vi "Init Incoming Single Point Signals.vi"(8 "error in":errorcluster, 11 "Incoming Single Point Configuraiton":T1 {"Channel Pairs"."Chan Refs" format="%.0x"}) -> (0 "error out":errorcluster, 3 "Incoming Single Point Configuraiton":T5 {"Channel Pairs"."Chan Refs" format="%.0x"})   [LabVIEW 2013, in "J1939 Addon Engine.lvlib"]
uses:
  J1939 Addon Engine.lvlib
  Types/Incoming Single Point Configuration.ctl
  Types/Incoming Single Point Frame Pairs.ctl
  Types/Incoming Single Point Channel Pairs.ctl
  <vilib>/NI Veristand/Custom Device API/Data Reference.ctl
  Shared/Types/SysDef Incoming Single Point Configurations.ctl
  Shared/Types/SysDef Incoming Frame Configuration.ctl
  <vilib>/xnet/xnet.llb/XNET Create Session (Conversion).vi
  <vilib>/NI Veristand/Custom Device API/Custom Device API.lvlib
  Shared/J1939 Addon Shared.lvlib
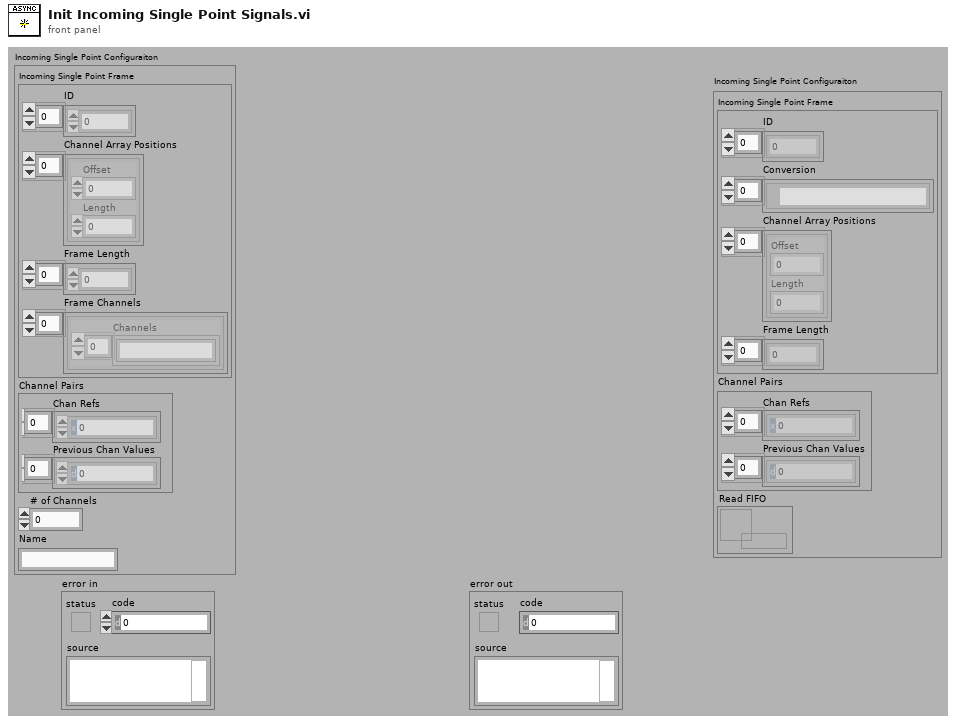
[diagram p1: front panel]
types:
  T1 = typedef "J1939 Addon Shared.lvlib/SysDef Incoming Single Point Configurations.ctl" = cluster{"Incoming Single Point Frame":T2, "Channel Pairs":T3, "# of Channels":u32, "Name":string}
  T2 = typedef "J1939 Addon Shared.lvlib/SysDef Incoming Frame Configuration.ctl" = cluster{"ID":u32[], "Channel Array Positions":cluster{"Offset":u32, "Length":u32}[], "Frame Length":u32[], "Frame Channels":cluster{"Channels":string[]}[]}
  T3 = typedef "J1939 Addon Engine.lvlib/Incoming Single Point Channel Pairs.ctl" = cluster{"Chan Refs":T4[], "Previous Chan Values":dbl[]}
  T4 = typedef "Custom Device API.lvlib/Data Reference.ctl" = i32
  T5 = typedef "J1939 Addon Engine.lvlib/Incoming Single Point Configuration.ctl" = cluster{"Incoming Single Point Frame":T6, "Channel Pairs":T3, "Read FIFO":refnum<k33>}
  T6 = typedef "J1939 Addon Engine.lvlib/Incoming Single Point Frame Pairs.ctl" = cluster{"ID":u32[], "Conversion":refnum<k21>[], "Channel Array Positions":cluster{"Offset":u32, "Length":u32}[], "Frame Length":u32[]}
  T7 = cluster{"read mode":enum16{"polling", "blocking"}, "write mode":enum16{"polling", "blocking"}}
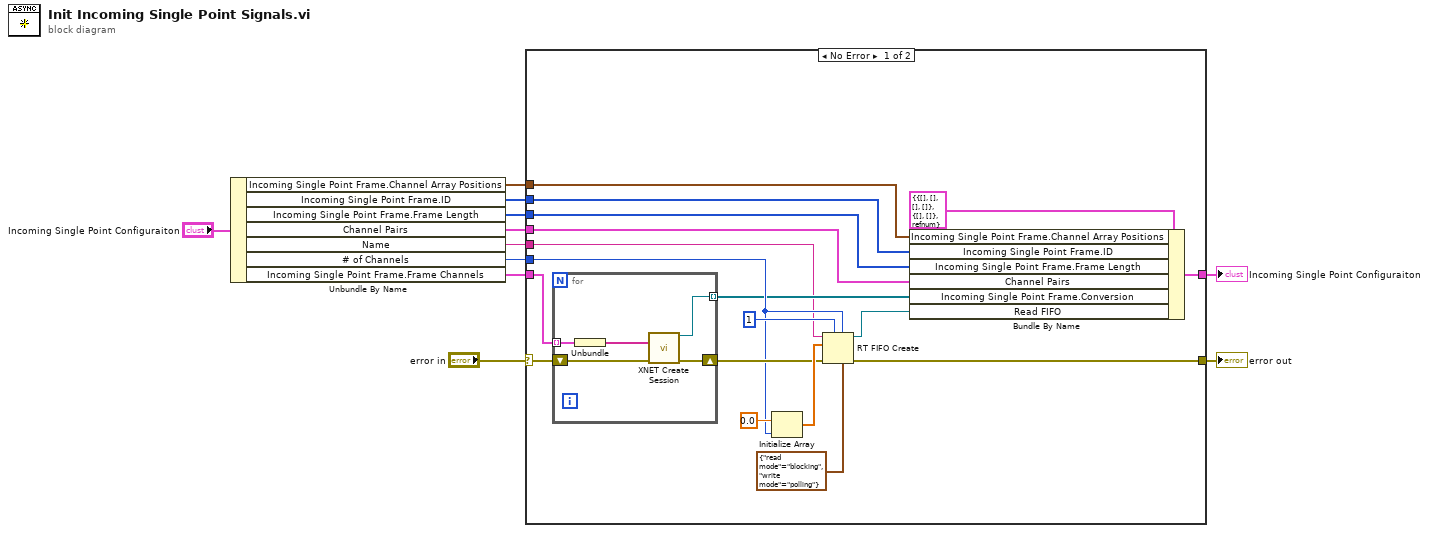
[diagram p0: block diagram]
diagram:
  n1 = Unbundle By Name("Incoming Single Point Configuraiton") -> ("Incoming Single Point Frame.Channel Array Positions"=w5:cluster{"Offset":u32, "Length":u32}[], "Incoming Single Point Frame.ID"=w4:u32[], "Incoming Single Point Frame.Frame Length"=w3:u32[], "Channel Pairs"=w2:T3, "Name"=w1:string, "# of Channels"=w6:u32, "Incoming Single Point Frame.Frame Channels"=w7:cluster{"Channels":string[]}[])
  n2 = case shown="No Error" "error in" {
    selector: "error in" -> [w20 w35]
    tunnel: [w27 _] -> w9
    tunnel: [w26 w35] -> w11
    tunnel: w7 -> [w21 _]
    tunnel: w6 -> [w18 _]
    tunnel: w5 -> [w17 _]
    tunnel: w4 -> [w16 _]
    tunnel: w3 -> [w15 _]
    tunnel: w2 -> [w14 _]
    tunnel: w1 -> [w12 _]
    frame No Error {
      n3 = for {
        tunnel: [w34] -> w13 mode=indexing
        tunnel: w21 -> [w33] mode=indexing
        shift-right: [w30] -> w19
        shift-left: w20 -> [w31]
        n4 = Unbundle(w33) -> ("Channels"=w32:string[])
        n5 = call-poly <vilib>:"XNET Create Session.vi"("signal list"=w32, "error in (no error)"=w31) -> ("session out"=w34:refnum<k21>, "error out"=w30:errorcluster)  [unwired: 12 in]
      }
      n6 = Initialize Array(0.0 ("element"), w18) -> (w25:dbl[])
      n7 = RT FIFO Create(0:w12, 1:w25, 3:w19, 4:u32 1 ("size (10)"), 6:w18, 7:T7 {"read mode"=enum."blocking", "write mode"=enum."polling"} ("r/w modes (polling,polling)")) -> (8:w23:refnum<k33>, 11:w26:errorcluster)  [unwired: 2 in, 1 out]
      n8 = Bundle By Name(cluster=T5 {"Incoming Single Point Frame"={"ID"=[], "Conversion"=[], "Channel Array Positions"=[], "Frame Length"=[]}, "Channel Pairs"={"Chan Refs"=[], "Previous Chan Values"=[]}, "Read FIFO"=refnum} ("Incoming Single Point Configuraiton"), "Incoming Single Point Frame.Channel Array Positions"=w17, "Incoming Single Point Frame.ID"=w16, "Incoming Single Point Frame.Frame Length"=w15, "Channel Pairs"=w14, "Incoming Single Point Frame.Conversion"=w13, "Read FIFO"=w23) -> (w27:T5)
    }
    frame Error {
    }
  }
  "error out" <- w11
  "Incoming Single Point Configuraiton" <- w9
